vi "GEOM_CommandSwitch.vi"(8 "error in (no error)":errorcluster, 10 "command in":string) -> (0 "error out":errorcluster, 1 "swhitches":string[](array[string]), 2 "command out":string, 4 "arguments":string[](array[string]))   [LabVIEW 2016]
panel:
  in  "num arguments":u16[](array[numeric])=[0, 0, 0, 0, 0, 0, 0, 0, 0, 0, 0, 0, 0, 0, 1]
  in  "switches":string[](array[string])=["-str", "-string", "-force", "-bin", "-clean", "-full", "-type", "-parse", "-all", "-raw", "-alarm", "-unit", "-params", "-list", "-detformat"]
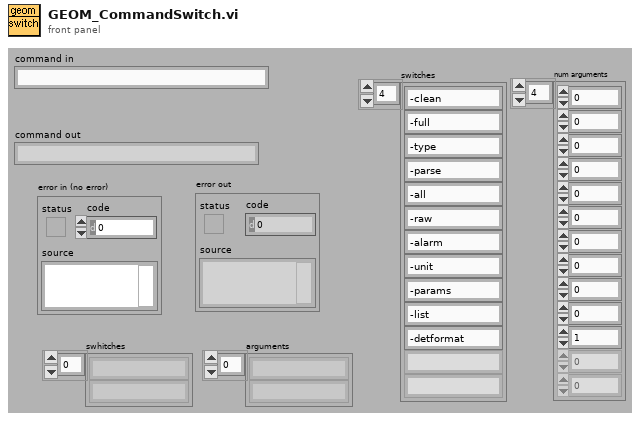
[diagram p1: front panel]
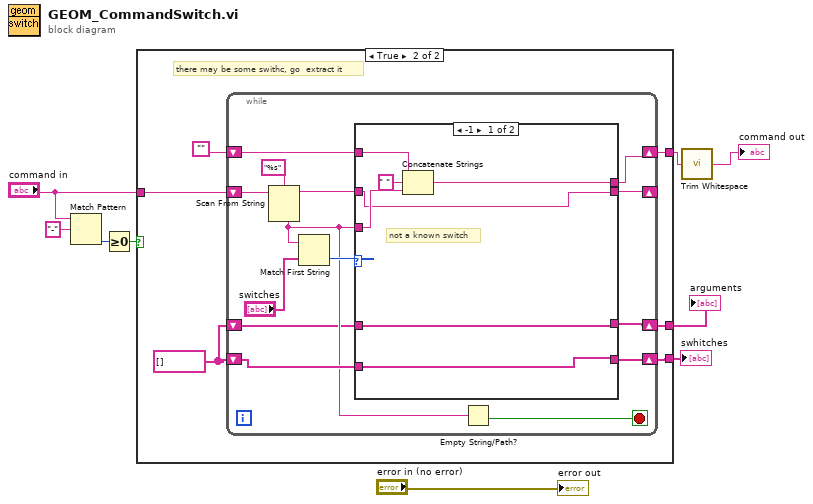
[diagram p0: block diagram]
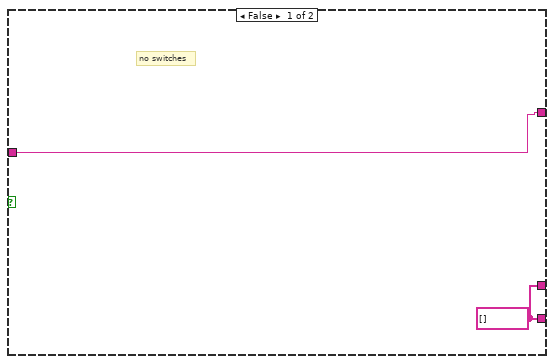
[diagram p2: hidden frame]
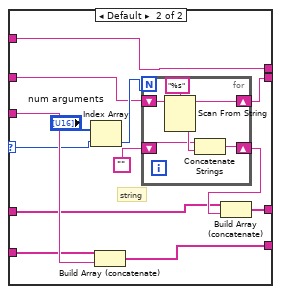
[diagram p3: hidden frame]
diagram:
  n1 = Match Pattern(string="command in", regular expression="-") -> (offset past match=w4:i32)  [unwired: 4 out]
  n2 = Greater Or Equal To 0?(x=w4) -> (x >= 0?=w3:bool)
  n3 = case shown="True" w3 {
    tunnel: "command in" -> [w11 w17]
    tunnel: [w10 w15] -> w9
    tunnel: [w11 w14] -> w8
    tunnel: [w10 w12] -> w1
    frame False {
      w10 = string[] []
      # "no switches"
    }
    frame True {
      w13 = string[] []
      # "there may be some swithc, go  extract it"
      n4 = while {
        shift-right: [w24] -> _
        shift-left: w17 -> [w31]
        shift-right: [w27] -> w14
        shift-left: "" -> [w26]
        shift-right: [w23] -> w15
        shift-left: w13 -> [w22]
        shift-right: [w19] -> w12
        shift-left: w13 -> [w18]
        stop <- w21 stop-if-true
        n5 = Scan From String(format string="%s", input string=w31) -> (remaining string=w25:string, output 1=w20:string)  [unwired: 2 in, 3 out]
        n6 = Match First String(2:"switches", 3:w20) -> (0:w28:i32)  [unwired: 1 out]
        n7 = case shown="-1" w28 {
          selector: w28 -> [_ w46]
          tunnel: [w38 w51] -> w27
          tunnel: w26 -> [w37 w51]
          tunnel: w20 -> [w35 w50]
          tunnel: w25 -> [w34 w44]
          tunnel: [w34 w39] -> w24
          tunnel: [w33 w49] -> w23
          tunnel: w22 -> [w33 w48]
          tunnel: [w32 w41] -> w19
          tunnel: w18 -> [w32 w40]
          frame -1 {
            # "not a known switch"
            n8 = Concatenate Strings(w37, " " ("string"), w35) -> (w38:string)
          }
          frame Default {
            # "string"
            n9 = Index Array(array="num arguments", index=w46) -> (element=w45:u16)
            n10 = Build Array (concatenate)(w48, w50) -> (w49:string[])
            n11 = for {
              N: w45 -> [_]
              shift-right: [w56] -> w39
              shift-left: w44 -> [w52]
              shift-right: [w54] -> w42
              shift-left: "" -> [w53]
              n12 = Scan From String(format string="%s", input string=w52) -> (remaining string=w56:string, output 1=w55:string)  [unwired: 2 in, 3 out]
              n13 = Concatenate Strings(w53, w55) -> (w54:string)
            }
            n14 = Build Array (concatenate)(w40, w42) -> (w41:string[])
          }
        }
        n15 = Empty String/Path?(string/path=w20) -> (empty?=w21:bool)
      }
    }
  }
  "swhitches" <- w9
  "arguments" <- w1
  n16 = call <vilib>:"Trim Whitespace.vi"("string"=w8) -> ("trimmed string"=→"command out":string)  [unwired: 1 in]
  "error out" <- "error in (no error)"
